vi "Main.vi"(10 "Acquisition Panel":refnum<vi>, 11 "Module Admin":refnum<class "Delacor_lib_QMH_Module Admin.lvclass">) -> ()   [LabVIEW 2020, in "Acquisition whit helper loop.lvlib"]
doc: "This template is based off of the Queued Message Handler design pattern and the Queued Message Handler project template that ships with LabVIEW.\n\nThe main difference is that the queue is private to this module and communication between modules is performed via Broadcast and Request events.\n\nRequest events are wrapped in public API methods and are handled in the Event Handling Loop (EHL) of this VI. Any module can register for Broadcast events sent by this module. The EHL generates messages based on user interface actions.\n\nThe Message Handling Loop (MHL) processes messages generated by the EHL, or by other messages. The messages are string values, so new messages can be added easily to the Message Cases case structure in the MHL. Each message cluster can also provide an optional value for Message Data, which is a variant that can be converted to whatever message-specific data is required.\n_____\nBased on Delacor QMH Project Template 5.0.0.82."
uses:
  Acquisition whit helper loop.lvlib
  <vilib>/Delacor/Delacor QMH/Libraries/Module Admin_class/Delacor_lib_QMH_Module Admin.lvclass
  Module Data--cluster.ctl
  Stop Helper Loop Argument--cluster.ctl
  <vilib>/Delacor/Delacor QMH/Libraries/Message Queue_class/Delacor_lib_QMH_Message Queue.lvclass/Delacor_lib_QMH_Message Queue.ctl
  Stop Argument--cluster.ctl
  <vilib>/Delacor/Delacor QMH/Libraries/Module Admin_class/Delacor_lib_QMH_Module Admin.lvclass/Delacor_lib_QMH_Module Admin.ctl
  <vilib>/Utility/miscctls.llb/LVPointTypeDef.ctl
  Start Acquisition Argument--cluster.ctl
  <vilib>/Delacor/Delacor QMH/Libraries/Message Queue_class/Delacor_lib_QMH_Enqueue Message (Single).vi
  <vilib>/Delacor/Delacor QMH/Libraries/Module Admin_class/Delacor_lib_QMH_Get External Launch.vi
  <vilib>/Utility/error.llb/Error Cluster From Error Code.vi
  <vilib>/ErrorRing/Error Ring.xnode
  <vilib>/Delacor/Delacor QMH/Libraries/Message Queue_class/Delacor_lib_QMH_Message Queue.lvclass
panel:
  out "current time":timestamp
  in  "Simulate MHL Error":bool
  in  "Simulate EHL Error":bool
  out "error out":errorcluster
  out "Status":string
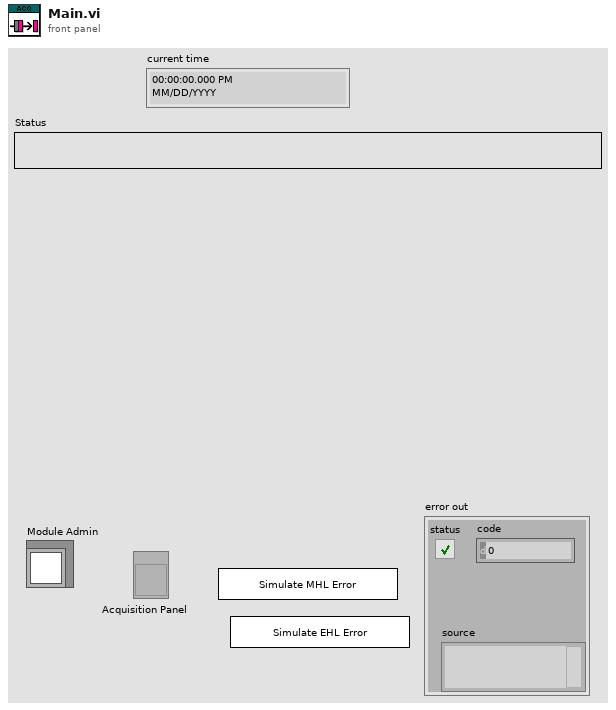
[diagram p1: front panel]
types:
  T1 = typedef "Acquisition whit helper loop.lvlib/Request Events--cluster.ctl" = cluster{"Stop Module":refnum<user-event>, "Show Panel":refnum<user-event>, "Hide Panel":refnum<user-event>, "Get Module Execution Status":refnum<user-event>, "Show Diagram":refnum<user-event>, "Start Helper Loop":refnum<user-event>, "Stop Helper Loop":refnum<user-event>}
  T2 = typedef "Acquisition whit helper loop.lvlib/Module Data--cluster.ctl" = cluster{"Status":string}
  T3 = enum32{"invalid lock state", "Not Locked", "Locked (No Password)", "Password-protected"}
  T4 = typedef "Acquisition whit helper loop.lvlib/Stop Argument--cluster.ctl" = cluster{"Origin":string, "Exit via Stop Module Req?":bool, "Wait for Module to stop?":bool}
  T5 = typedef "LVPointTypeDef.ctl" = cluster{"Horizontal":i16, "Vertical":i16}
  T6 = enum32{"Invalid", "Standard", "Closed", "Hidden", "Minimized", "Maximized"}
  T7 = typedef "Start Acquisition Argument--cluster.ctl" = cluster{"Boolean":bool}
  T8 = typedef "Acquisition whit helper loop.lvlib/Stop Helper Loop Argument--cluster.ctl" = cluster{"Boolean":bool}
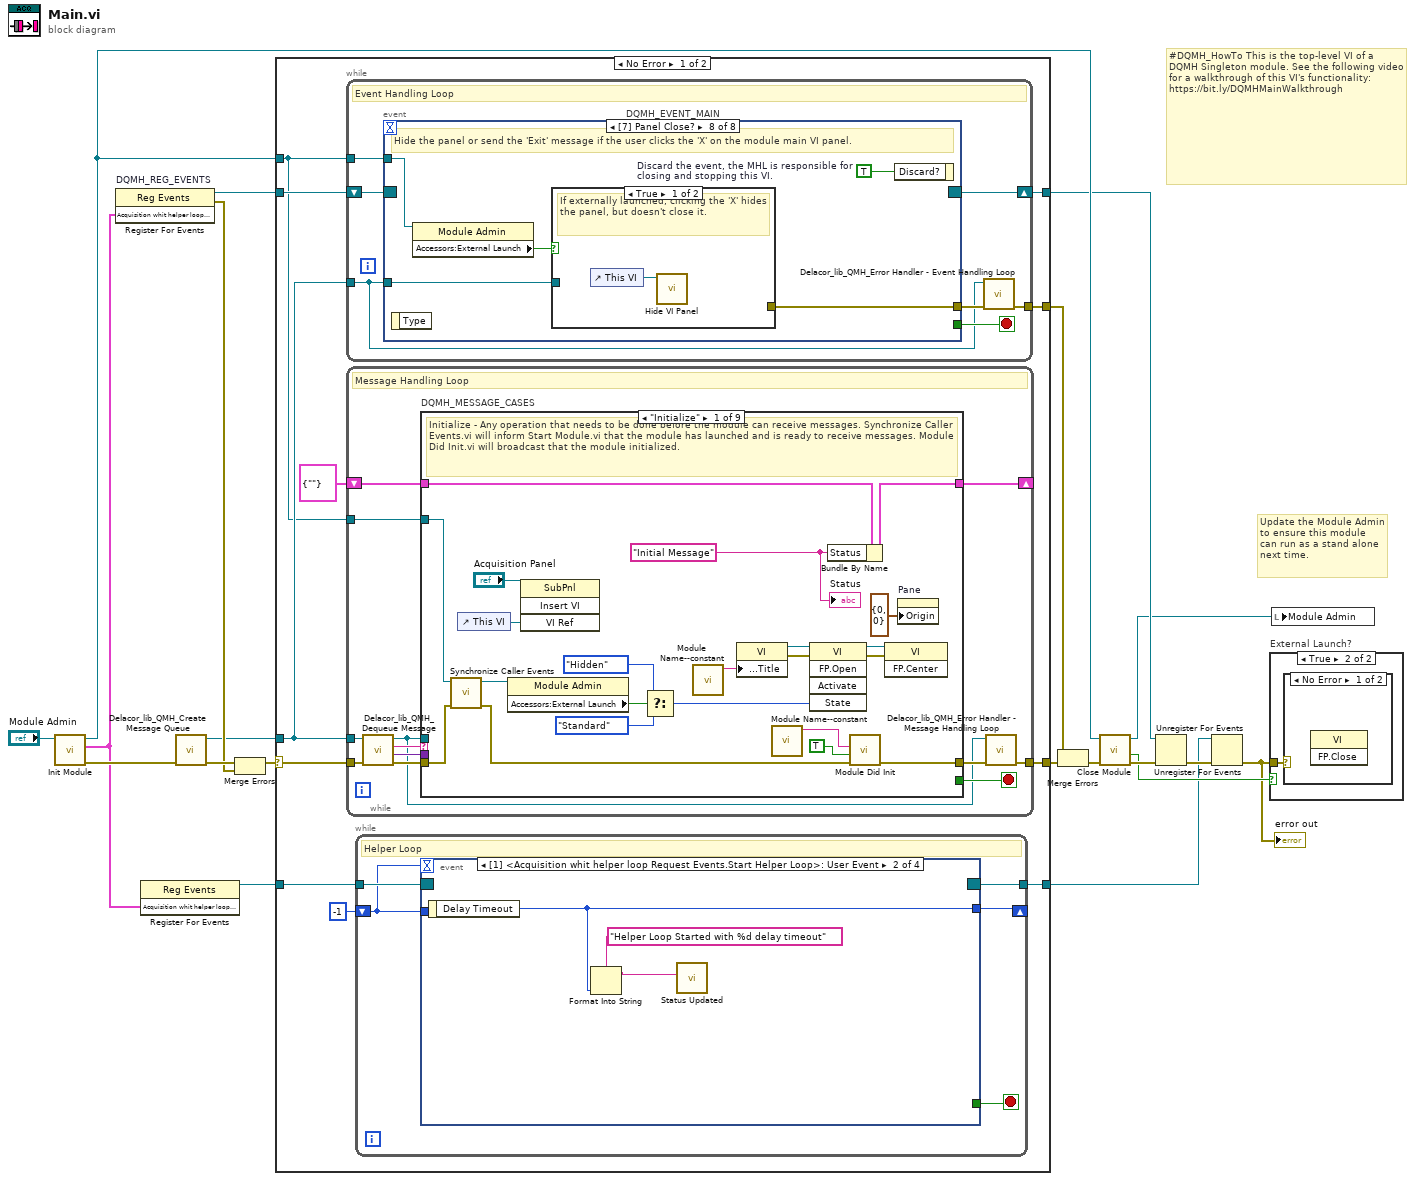
[diagram p0: block diagram]
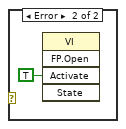
[diagram p3: hidden frame]
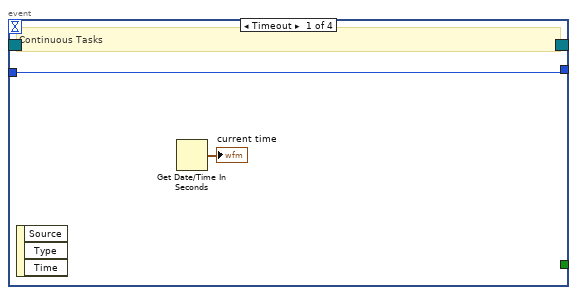
[diagram p4: hidden frame]
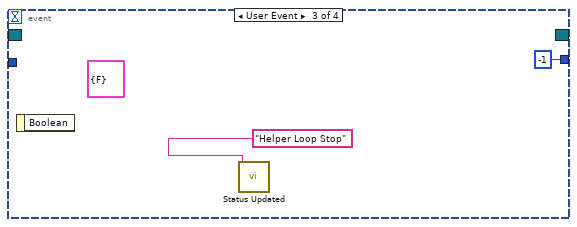
[diagram p5: hidden frame]
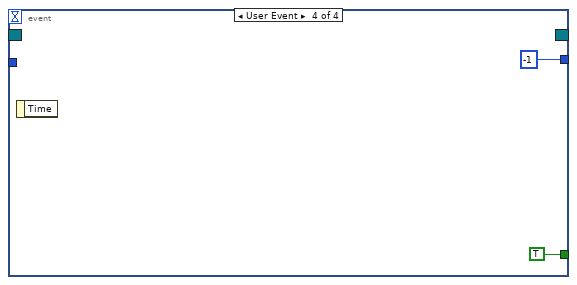
[diagram p6: hidden frame]
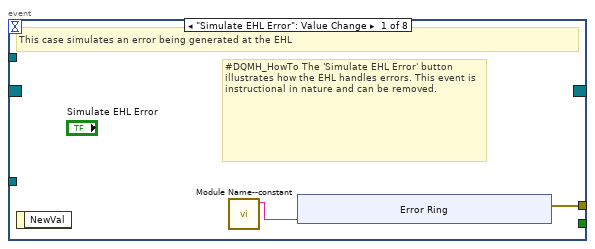
[diagram p7: hidden frame]
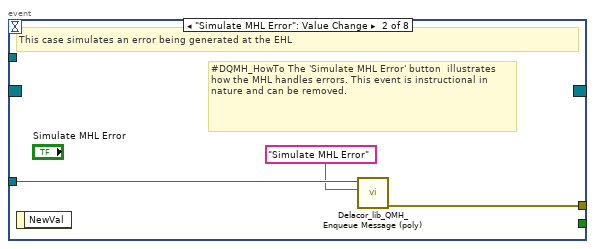
[diagram p8: hidden frame]
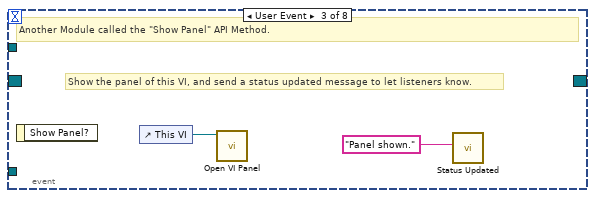
[diagram p9: hidden frame]
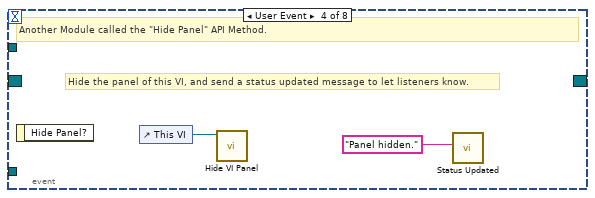
[diagram p10: hidden frame]
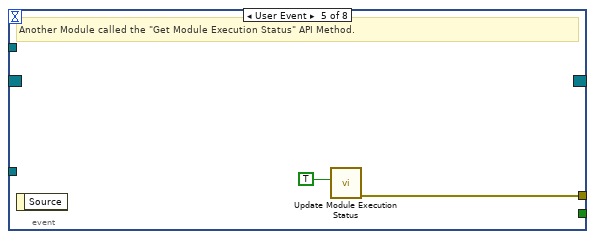
[diagram p11: hidden frame]
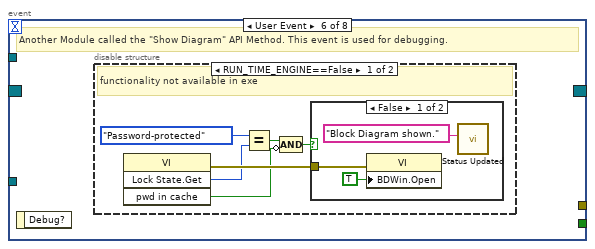
[diagram p12: hidden frame]
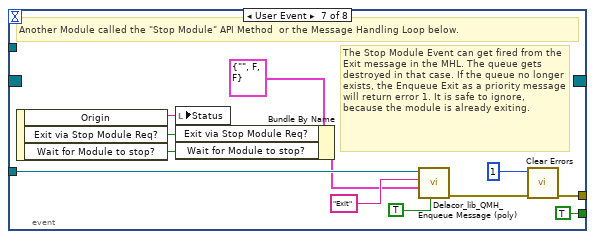
[diagram p15: hidden frame]
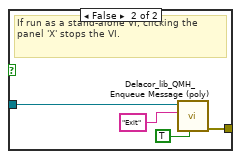
[diagram p16: hidden frame]
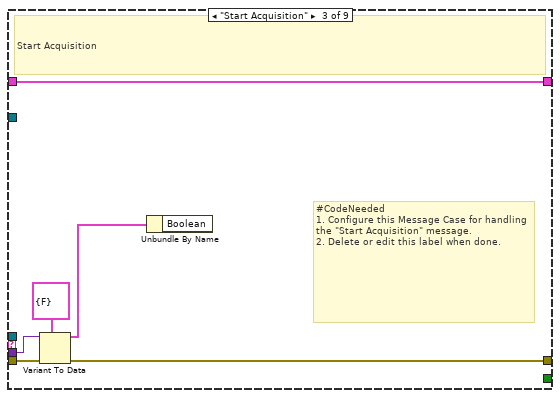
[diagram p18: hidden frame]
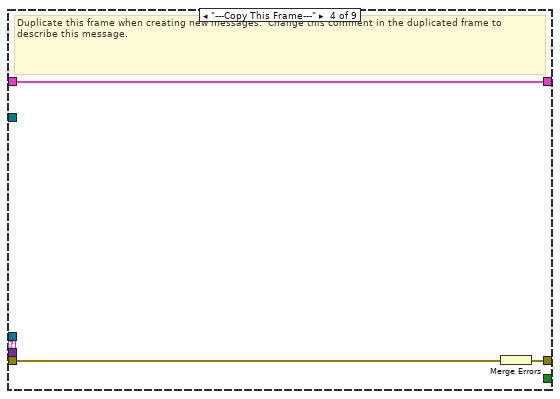
[diagram p19: hidden frame]
diagram:
  # "#DQMH_HowTo This is the top-level VI of a DQMH Singleton module. See the following video for a walkthrough of this VI's functionality: https://bit.ly/DQMHMainWalkthrough"
  # "Update the Module Admin to ensure this module can run as a stand alone next time."
  n1 = call "Init Module.vi"("Singleton Module Admin in"="Module Admin") -> ("error out"=w19:errorcluster, "Acquisition whit helper loop Request Events"=w3:T1, "Singleton Module Admin out"=w11:refnum<class "Delacor_lib_QMH_Module Admin.lvclass">)  [unwired: 8 in]
  n2 = register-events "DQMH_REG_EVENTS"(w3) -> (reference out=w9:refnum<event-registration>, error out=w12:errorcluster)  [unwired: 2 in]
  n3 = register-events(w3) -> (reference out=w4:refnum<event-registration>)  [unwired: 2 in, 1 out]
  n4 = call <vilib>:"Delacor_lib_QMH_Create Message Queue.vi"("error in (no error)"=w19) -> ("error out"=w14:errorcluster, "Message Queue"=w8:refnum<class "Delacor_lib_QMH_Message Queue.lvclass">)  [unwired: 9 in]
  n5 = Merge Errors(w14, w12) -> (w13:errorcluster)
  n6 = case shown="No Error" w13 {
    selector: w13 -> [w29 w210]
    tunnel: [w31 w209] -> w20
    tunnel: [w28 w215] -> w10
    tunnel: w9 -> [w26 w215]
    tunnel: w8 -> [w25 w208]
    tunnel: [w30 _] -> w17
    tunnel: w11 -> [w24 w211]
    tunnel: w4 -> [w23 w207]
    tunnel: [w22 w207] -> w1
    frame No Error {
      n7 = while {
        tunnel: w25 -> [w46]
        shift-right: [w49] -> w28
        shift-left: w26 -> [w50]
        tunnel: [w51] -> w30
        tunnel: w24 -> [w47]
        stop <- w48 stop-if-true
        # "Event Handling Loop"
        n8 = event "DQMH_EVENT_MAIN" shown="[7] Panel Close?" {
          selector: w50 -> [_ _ _ _ _ _ _ _]
          dyn-events: [_ _ _ _ _ _ _ _] -> w49
          timeout: _ -> [_ _ _ _ _ _ _ _]
          tunnel: [_ _ _ _ _ _ TRUE ("Discard?") _] -> w48
          tunnel: w46 -> [_ w63 _ _ _ _ w87 w94]
          tunnel: [w54 w64 _ _ w70 _ w90 w96] -> w52
          tunnel: w47 -> [_ _ _ _ _ _ _ w93]
          event "Simulate EHL Error": Value Change {
            # "#DQMH_HowTo The 'Simulate EHL Error' button  illustrates how the EHL handles errors. This event is instructional in nature and can be removed."
            # "This case simulates an error being generated at the EHL"
            n9 = event-data() -> ()  [unwired: 1 in, 1 out]
            n10 = call "Module Name--constant.vi"() -> ("Module Name"=w53:string)  [unwired: 11 in]
            n11 = xnode "Error Ring"("parameter 0"=w53) -> ("error out"=w54:errorcluster)
          }
          event "Simulate MHL Error": Value Change {
            # "#DQMH_HowTo The 'Simulate MHL Error' button  illustrates how the MHL handles errors. This event is instructional in nature and can be removed."
            # "This case simulates an error being generated at the EHL"
            n12 = event-data() -> ()  [unwired: 1 in, 1 out]
            n13 = call-poly <vilib>:"Delacor_lib_QMH_Enqueue Message (poly).vi"("Message"="Simulate MHL Error", "Message Queue in"=w63) -> ("error out"=w64:errorcluster)  [unwired: 8 in, 1 out]
          }
          event User Event {
            # "Show the panel of this VI, and send a status updated message to let listeners know."
            # "Another Module called the \"Show Panel\" API Method."
            n14 = event-data() -> ()  [unwired: 1 in, 1 out]
            n15 = control-ref of="This VI"() -> (w66:refnum<vi>)
            n16 = call "Open VI Panel.vi"("VI"=w66) -> ()  [unwired: 10 in, 1 out]
            n17 = call "Status Updated.vi"("Status"="Panel shown." ("format string")) -> ()  [unwired: 10 in, 1 out]
          }
          event User Event {
            # "Hide the panel of this VI, and send a status updated message to let listeners know."
            # "Another Module called the \"Hide Panel\" API Method."
            n18 = event-data() -> ()  [unwired: 1 in, 1 out]
            n19 = control-ref of="This VI"() -> (w68:refnum<vi>)
            n20 = call "Hide VI Panel.vi"("VI"=w68) -> ()  [unwired: 10 in, 1 out]
            n21 = call "Status Updated.vi"("Status"="Panel hidden." ("format string")) -> ()  [unwired: 10 in, 1 out]
          }
          event User Event {
            # "Another Module called the \"Get Module Execution Status\" API Method."
            n22 = event-data() -> ()  [unwired: 1 in, 1 out]
            n23 = call "Update Module Execution Status.vi"("Running?"=TRUE) -> ("error out"=w70:errorcluster)  [unwired: 10 in]
          }
          event User Event {
            # "Another Module called the \"Show Diagram\" API Method. This event is used for debugging."
            n24 = event-data() -> ()  [unwired: 1 in, 1 out]
            n25 = disable-structure shown="RUN_TIME_ENGINE==False" {
              frame condition #0 (active) {
                # "functionality not available in exe"
                n26 = invoke class="VI" method="Lock State.Get"() -> (error out=w76:errorcluster, "Get Lock State"=w75:T3, "pwd in cache"=w72:bool)  [unwired: 4 in, 1 out]
                n27 = Equal?(x=T3."Password-protected", y=w75) -> (x = y?=w73:bool)
                n28 = Compound Arithmetic op=AND(w73, invert w72) -> (w71:bool)
                n29 = case shown="False" w71 {
                  tunnel: w76 -> [w79 _]
                  frame False {
                    n30 = property class="VI"(error in=w79, "BDWin.Open"=TRUE ("Block Diagram Window:Open")) -> ()  [unwired: 1 in, 2 out]
                    n31 = call "Status Updated.vi"("Status"="Block Diagram shown." ("format string")) -> ()  [unwired: 10 in, 1 out]
                  }
                  frame True {
                    # "Password-protected VI, and the password is not in the cache. Do not show the diagram."
                  }
                }
              }
              frame condition #1 {
              }
            }
          }
          event User Event {
            # "The Stop Module Event can get fired from the Exit message in the MHL. The queue gets destroyed in that case. If the queue no longer exists, the Enqueue Exit as a priority message will return error 1. It is safe to ignore, because the module is already exiting."
            # "Another Module called the \"Stop Module\" API Method  or the Message Handling Loop below."
            n32 = event-data() -> ("Origin"=w86:string, "Exit via Stop Module Req?"=w82:bool, "Wait for Module to stop?"=w81:bool)  [unwired: 1 in]
            n33 = local write "Status"(w86) -> ()
            n34 = Bundle By Name(cluster=T4 {"Origin"="", "Exit via Stop Module Req?"=FALSE, "Wait for Module to stop?"=FALSE} ("Stop Argument"), "Exit via Stop Module Req?"=w82, "Wait for Module to stop?"=w81) -> (w80:T4)
            n35 = call-poly <vilib>:"Delacor_lib_QMH_Enqueue Message (poly).vi"("Priority Message? (F)"=TRUE, "Message Data"=w80, "Message"="Exit", "Message Queue in"=w87) -> ("error out"=w91:errorcluster)  [unwired: 6 in, 1 out]
            n36 = call <vilib>:"Clear Errors.vi"("error in (no error)"=w91, "specific error code to clear (0: all)"=1) -> ("error out"=w90:errorcluster)  [unwired: 4 in, 1 out]
          }
          event Panel Close? {
            w95 = TRUE  # Discard the event, the MHL is responsible for closing and stopping this VI.
            # "Hide the panel or send the 'Exit' message if the user clicks the 'X' on the module main VI panel."
            n37 = event-data() -> ()  [unwired: 1 in, 1 out]
            n38 = property class="Module Admin"(reference=w93) -> ("Accessors:External Launch"=w92:bool)  [unwired: 1 in, 2 out]
            n39 = case shown="True" w92 {
              tunnel: w94 -> [_ w100]
              tunnel: [_ w101] -> w96
              frame True {
                # "If externally launched, clicking the 'X' hides the panel, but doesn't close it."
                n40 = control-ref of="This VI"() -> (w97:refnum<vi>)
                n41 = call "Hide VI Panel.vi"("VI"=w97) -> ()  [unwired: 10 in, 1 out]
              }
              frame False {
                # "If run as a stand-alone VI, clicking the panel 'X' stops the VI."
                n42 = call-poly <vilib>:"Delacor_lib_QMH_Enqueue Message (poly).vi"("Priority Message? (F)"=TRUE, "Message"="Exit", "Message Queue in"=w100) -> ("error out"=w101:errorcluster)  [unwired: 7 in, 1 out]
              }
            }
            n43 = event-data("Discard?"=w95) -> ()  [unwired: 1 in, 1 out]
          }
        }
        n44 = call-dynamic "Delacor_lib_QMH_Error Handler - Event Handling Loop.vi"("error in (no error)"=w52, "Message Queue in"=w46) -> ("dup error in"=w51:errorcluster)  [unwired: 8 in, 1 out]
      }
      n45 = while {
        tunnel: w25 -> [w104]
        shift-right: [w108] -> _
        shift-left: T2 {"Status"=""} ("Data Cluster") -> [w109]
        tunnel: w29 -> [w112]
        tunnel: [w110] -> w31
        tunnel: w24 -> [w102]
        stop <- w107 stop-if-true
        # "Message Handling Loop"
        n46 = call-dynamic "Delacor_lib_QMH_Dequeue Message.vi"("error in (no error)"=w112, "Message Queue in"=w104) -> ("error out"=w111:errorcluster, "Message Data"=w105:variant, "Message"=w106:string, "Message Queue out"=w103:refnum<class "Delacor_lib_QMH_Message Queue.lvclass">)  [unwired: 6 in]
        n47 = case "DQMH_MESSAGE_CASES" shown="\"Initialize\"" w106 {
          selector: w106 -> [_ _ _ _ _ _ _ _ w194]
          tunnel: w103 -> [_ _ _ _ _ _ w164 w186 _]
          tunnel: w111 -> [w133 w137 w143 w146 w148 w153 w171 w192 w196]
          tunnel: [w131 w137 w141 w145 w148 w152 w167 w189 w197] -> w113
          tunnel: w109 -> [w122 w136 w142 w144 w147 w150 w166 w185 w195]
          tunnel: [w121 w136 w142 w144 w147 w150 w166 w185 w195] -> w108
          tunnel: [_ _ _ _ _ _ _ w184 _] -> w107
          tunnel: w105 -> [_ _ w140 _ _ _ w165 w183 _]
          tunnel: w102 -> [w123 _ _ _ _ _ w163 w178 _]
          frame "Initialize" {
            w116 = "Initial Message" ("Initial Message")
            # "Initialize - Any operation that needs to be done before the module can receive messages. Synchronize Caller Events.vi will inform Start Module.vi that the module has launched and is ready to receive messages. Module Did Init.vi will broadcast that the module initialized."
            n48 = call "Synchronize Caller Events.vi"("error in (no error)"=w133, "Singleton Module Admin in"=w123) -> ("error out"=w132:errorcluster, "Singleton Module Admin out"=w118:refnum<class "Delacor_lib_QMH_Module Admin.lvclass">)  [unwired: 8 in]
            n49 = control-ref of="This VI"() -> (w114:refnum<vi>)
            n50 = property class="Module Admin"(reference=w118) -> ("Accessors:External Launch"=w127:bool)  [unwired: 1 in, 2 out]
            n51 = invoke class="SubPnl" method="Insert VI"(reference="Acquisition Panel", "VI Ref"=w114) -> ()  [unwired: 2 in, 4 out]
            n52 = Select(t=T6."Hidden" ("State"), s=w127, f=T6."Standard" ("State")) -> (s? t:f=w124:T6)
            n53 = call "Module Name--constant.vi"() -> ("Module Name"=w130:string)  [unwired: 11 in]
            n54 = property class="VI"("Front Panel.Title"=w130) -> (reference out=w129:refnum<vi>, error out=w135:errorcluster)  [unwired: 2 in]
            n55 = call "Module Name--constant.vi"() -> ("Module Name"=w119:string)  [unwired: 11 in]
            n56 = invoke class="VI" method="FP.Open"(reference=w129, error in=w135, "State"=w124) -> (reference out=w128:refnum<vi>, error out=w134:errorcluster)  [unwired: 2 in, 3 out]
            n57 = Bundle By Name(cluster=w122, "Status"=w116) -> (w121:T2)
            n58 = call "Module Did Init.vi"("error in (no error)"=w132, "Initialized?"=TRUE, "Origin"=w119) -> ("error out"=w131:errorcluster)  [unwired: 8 in]
            n59 = invoke class="VI" method="FP.Center"(reference=w128, error in=w134) -> ()  [unwired: 1 in, 3 out]
            n60 = property on="Pane" class="Pane"("Origin"=T5 {"Horizontal"=0, "Vertical"=0}) -> ()  [unwired: 2 in, 2 out]
            "Status" <- w116
          }
          frame "--- Module Specific ---" {
            # "Separator -- The following cases handle messages specific to this Module."
          }
          frame "Start Acquisition" {
            # "#CodeNeeded\n1. Configure this Message Case for handling the \"Start Acquisition\" message.\n2. Delete or edit this label when done."
            # "Start Acquisition"
            n61 = Variant To Data(error in=w143, type=T7 {"Boolean"=FALSE} ("Start Acquisition Argument"), Variant=w140) -> (data=w138:T7, error out=w141:errorcluster)
            n62 = Unbundle By Name(w138) -> ()  [unwired: 1 out]
          }
          frame "---Copy This Frame---" {
            # "Duplicate this frame when creating new messages.  Change this comment in the duplicated frame to describe this message."
            n63 = Merge Errors(w146) -> (w145:errorcluster)
          }
          frame "--- Exit and Error Handling---" {
            # "Separator - The following cases handle errors and exit messages."
          }
          frame "Simulate MHL Error" {
            # "#DQMH_HowTo The 'Simulate MHL Error' button  illustrates how the MHL handles errors. This event is instructional in nature and can be removed."
            # "Simulate an error occurring at the MHL"
            n64 = call "Module Name--constant.vi"() -> ("Module Name"=w149:string)  [unwired: 11 in]
            n65 = xnode "Error Ring"("parameter 0"=w149) -> ("error out"=w151:errorcluster)
            n66 = Merge Errors(w153, w151) -> (w152:errorcluster)
          }
          frame "Error" {
            # "#CodeRecommended - If you ever change the name of this \"Error\" message, you'll need to update the name in the Check Loop Error.vi as well."
            # "#CodeRecommended - If the module is running in standalone mode (External Launch = FALSE), this code will pop up an error dialog and call the 'Exit' message if an error occurs. Add more fine-grained error handling here."
            # "Error - Check the error message data and respond accordingly. This message is sent by the \"Error Handler\" VIs at the end of each loop in this application."
            n67 = property class="Module Admin"(reference=w163) -> ("Accessors:External Launch"=w162:bool)  [unwired: 1 in, 2 out]
            n68 = Variant To Data(error in=w171, type=errorcluster {"status"=FALSE, "code"=0, "source"=""} ("error constant"), Variant=w165) -> (data=w172:errorcluster, error out=w169:errorcluster)
            n69 = call "Module Name--constant.vi"() -> ("Module Name"=w161:string)  [unwired: 11 in]
            n70 = call "Error Reported.vi"("Additional Information"=w161, "Error"=w172) -> ()  [unwired: 9 in, 1 out]
            n71 = case shown="False" w162 {
              tunnel: [w177 _] -> w168
              tunnel: w164 -> [w175 _]
              tunnel: w172 -> [w176 _]
              frame False {
                # "If the module is running standalone, then pop up an error dialog and call the \"Exit\" message."
                n72 = call <vilib>:"Simple Error Handler.vi"("error in (no error)"=w176) -> ()  [unwired: 4 in, 5 out]
                n73 = call-poly <vilib>:"Delacor_lib_QMH_Enqueue Message (poly).vi"("Priority Message? (F)"=TRUE, "Message"="Exit", "Message Queue in"=w175) -> ("error out"=w177:errorcluster)  [unwired: 7 in, 1 out]
              }
              frame True {
                # "If the module was launched externally, calling the Error Reported broadcast VI is the only action performed by the \"Error\" message. The module's caller can then process the error appropriately."
              }
            }
            n74 = Merge Errors(w169, w168) -> (w167:errorcluster)
            n75 = local write "error out"(w167) -> ()
          }
          frame "Exit" {
            w182 = 91  # 91: not all Exit messages will have an argument
            w184 = TRUE  # Stop the VI
            # "Release the message queue reference"
            # "#CodeNeeded - Add any required cleanup code here"
            # "Exit - Exit the application."
            n76 = Variant To Data(error in=w192, type=T4 {"Origin"="", "Exit via Stop Module Req?"=FALSE, "Wait for Module to stop?"=FALSE} ("Stop Argument"), Variant=w183) -> (data=w180:T4, error out=w188:errorcluster)
            n77 = call <vilib>:"Clear Errors.vi"("error in (no error)"=w188, "specific error code to clear (0: all)"=w182) -> ("error out"=w191:errorcluster)  [unwired: 4 in, 1 out]
            n78 = control-ref of="This VI"() -> (w179:refnum<vi>)
            n79 = call-dynamic "Delacor_lib_QMH_Release Message Queue.vi"("error in (no error)"=w191, "Message Queue"=w186) -> ("error out"=w190:errorcluster)  [unwired: 9 in]
            n80 = call "Handle Exit.vi"("Stop Argument"=w180, "Admin in"=w178, "VI reference"=w179) -> ("error out"=w187:errorcluster)  [unwired: 7 in, 1 out]
            n81 = Merge Errors(w190, w187) -> (w189:errorcluster)
          }
          frame Default {
            # "'Default' case only runs if there is a message that isn't defined in any of the other cases.  Output a programming error."
            n82 = call "Module Name--constant.vi"() -> ("Module Name"=w193:string)  [unwired: 11 in]
            n83 = xnode "Error Ring"("parameter 0"=w194, "parameter 1"=w193) -> ("error out"=w198:errorcluster)
            n84 = Merge Errors(w196, w198) -> (w197:errorcluster)
          }
        }
        n85 = call-dynamic "Delacor_lib_QMH_Error Handler - Message Handling Loop.vi"("error in (no error)"=w113, "Message Queue in"=w103) -> ("dup error in"=w110:errorcluster)  [unwired: 8 in, 1 out]
      }
      n86 = while {
        tunnel: w23 -> [w36]
        tunnel: [w35] -> w22
        shift-right: [w34] -> _
        shift-left: -1 -> [w33]
        stop <- w32 stop-if-true
        # "Helper Loop"
        n87 = event shown="[1] <Acquisition whit helper loop Request Events.Start Helper Loop>: User Event" {
          selector: w36 -> [_ _ _ _]
          dyn-events: [_ _ _ _] -> w35
          timeout: w33 -> [_ _ _ _]
          tunnel: [w38 w39 -1 -1] -> w34
          tunnel: w33 -> [w38 _ _ _]
          tunnel: [_ _ _ TRUE] -> w32
          event Timeout {
            # "Continuous Tasks"
            n88 = event-data() -> ()  [unwired: 1 in, 3 out]
            n89 = Get Date/Time In Seconds() -> (seconds since 1Jan1904=→"current time":timestamp)
          }
          event User Event {
            n90 = event-data() -> ("Delay Timeout"=w39:i32)  [unwired: 1 in]
            n91 = Format Into String(format string="Helper Loop Started with %d delay timeout", w39) -> (resulting string=w41:string)  [unwired: 2 in, 1 out]
            n92 = call "Status Updated.vi"("Status"=w41) -> ()  [unwired: 10 in, 1 out]
          }
          event User Event {
            (unwired) T8 {"Boolean"=FALSE} ("Stop Helper Loop Argument")
            n93 = event-data() -> ()  [unwired: 1 in, 1 out]
            n94 = call "Status Updated.vi"("Status"="Helper Loop Stop" ("format string")) -> ()  [unwired: 10 in, 1 out]
          }
          event User Event {
            n95 = event-data() -> ()  [unwired: 1 in, 1 out]
          }
        }
      }
    }
    frame Error {
      # "Synchronize Caller Events.vi will inform Start Module.vi that the module has launched and will let the code calling Start Module.vi register for broadcasts and would permit the caller receive the broadcast that an error occurred at launch time."
      n96 = call-dynamic "Delacor_lib_QMH_Release Message Queue.vi"("error in (no error)"=w210, "Message Queue"=w208) -> ("error out"=w209:errorcluster)  [unwired: 9 in]
      n97 = call "Synchronize Caller Events.vi"("Singleton Module Admin in"=w211) -> ("error out"=w216:errorcluster)  [unwired: 9 in, 1 out]
      n98 = call "Module Name--constant.vi"() -> ("Module Name"=w214:string)  [unwired: 11 in]
      n99 = Format Into String(format string="An error occurred during initialization. %s is no longer running.", w214) -> (resulting string=w212:string)  [unwired: 2 in, 1 out]
      n100 = Merge Errors(w209, w216) -> (w217:errorcluster)
      n101 = call "Error Reported.vi"("Additional Information"=w212, "Error"=w217) -> ()  [unwired: 9 in, 1 out]
    }
  }
  n102 = Merge Errors(w17, w20) -> (w16:errorcluster)
  n103 = call "Close Module.vi"("error in (no error)"=w16, "Module Admin in"=w11) -> ("error out"=w18:errorcluster, "External Launch"=w5:bool, "Module Admin out"=w6:refnum<class "Delacor_lib_QMH_Module Admin.lvclass">)  [unwired: 7 in]
  n104 = Unregister For Events(event registration refnum=w10, error in=w18) -> (error out=w15:errorcluster)
  n105 = Unregister For Events(event registration refnum=w1, error in=w15) -> (error out=w2:errorcluster)
  "error out" <- w2
  n106 = case "External Launch?" shown="True" w5 {
    tunnel: w2 -> [_ w218]
    frame False {
    }
    frame True {
      n107 = case shown="No Error" w218 {
        frame No Error {
          n108 = invoke class="VI" method="FP.Close"() -> ()  [unwired: 3 in, 3 out]
        }
        frame Error {
          n109 = invoke class="VI" method="FP.Open"("Activate"=TRUE ("Activate?")) -> ()  [unwired: 4 in, 5 out]
        }
      }
    }
  }
  n110 = local write "Module Admin"(w6) -> ()
